vi "Bkgnd_place_names.vi"(1 "Numeric":i32) -> (0 "Array":string[](array[string]))   [LabVIEW 2017]
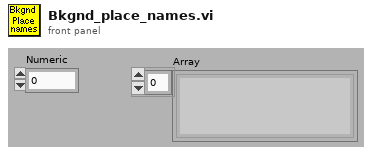
[diagram p1: front panel]
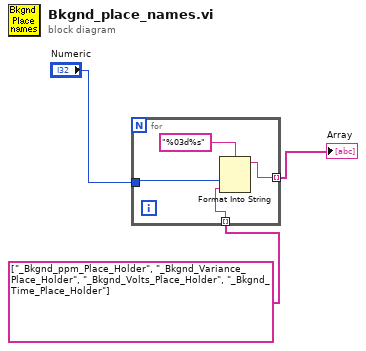
[diagram p0: block diagram]
diagram:
  n1 = for {
    tunnel: string[] ["_Bkgnd_ppm_Place_Holder", "_Bkgnd_Variance_Place_Holder", "_Bkgnd_Volts_Place_Holder", "_Bkgnd_Time_Place_Holder"] -> [w7] mode=indexing
    tunnel: [w5] -> w3 mode=indexing
    tunnel: "Numeric" -> [w6]
    n2 = Format Into String(format string="%03d%s", w6, w7) -> (resulting string=w5:string)  [unwired: 2 in, 1 out]
  }
  "Array" <- w3
